vi "RSNRPZctrl.vi"(0 "VISA session in":refnum<visa-resource-name> caption="VISA resource name", 1 "Resource Name (USB::0x0aad::0x000b::100000)":string="USB::0x0aad::0x00a7::101568", 5 "RSNPRZsettings":T1 caption="Settings :", 11 "error in (no error)":errorcluster, 12 "action":enum16{"close", "update", "read", "init"}(ring)) -> (4 "dup VISA session out":refnum<visa-resource-name> caption="VISA resource name", 6 "Measurement":dbl format="%.3p", 8 "connection status":bool, 15 "error out":errorcluster)   [LabVIEW 2019]
uses:
  RSNRPZcontrol.ctl
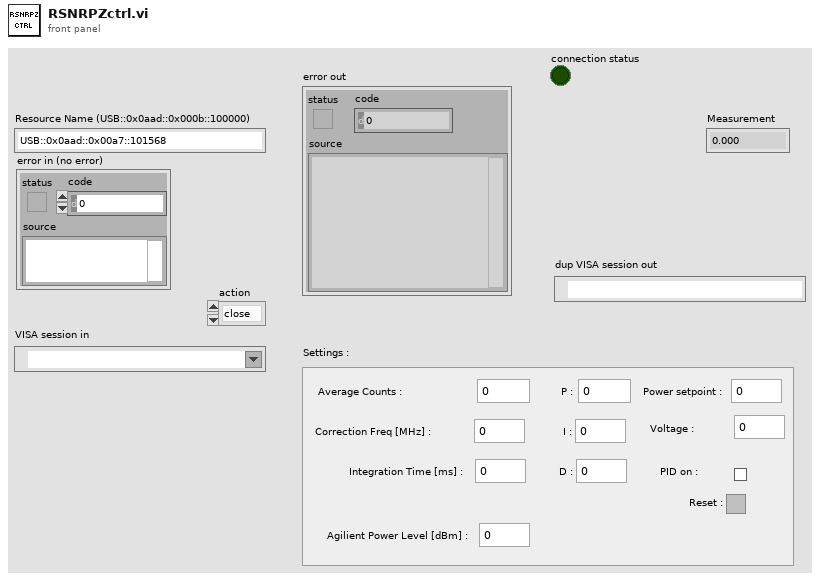
[diagram p1: front panel]
types:
  T1 = typedef "RSNRPZcontrol.ctl" = cluster{"Average Counts :":dbl, "Correction Freq [MHz] :":dbl, "Integration Time [ms] : ":dbl, "P :":dbl, "I :":dbl, "D :":dbl, "Power setpoint :":dbl, "PID on :":bool, "Voltage :":dbl, "Reset :":bool, "Agilient Power Level [dBm] :":dbl}
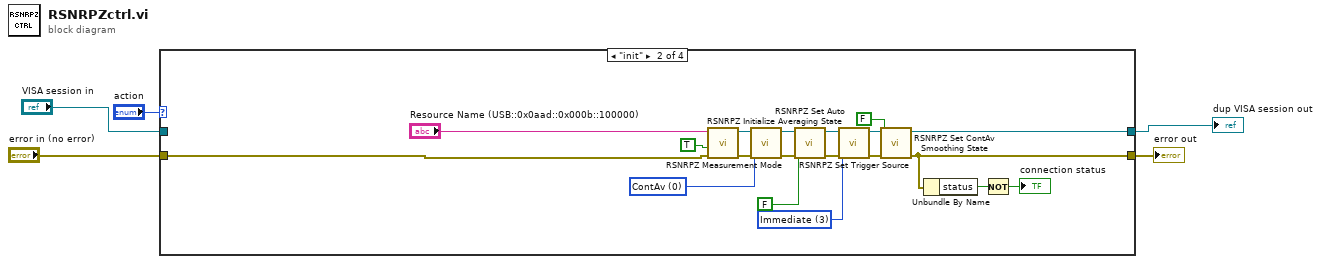
[diagram p0: block diagram]
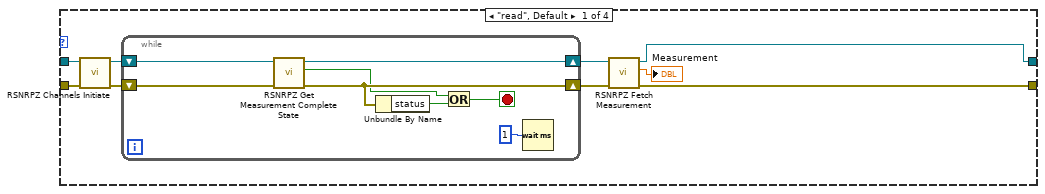
[diagram p2: hidden frame]
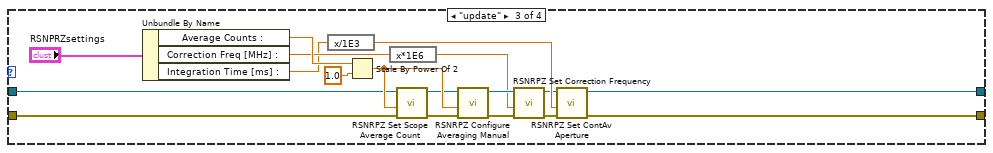
[diagram p3: hidden frame]
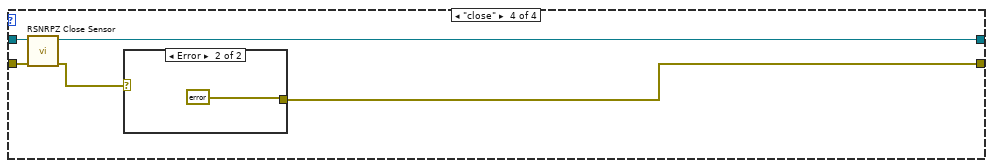
[diagram p4: hidden frame]
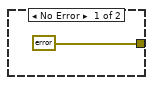
[diagram p5: hidden frame]
diagram:
  n1 = case shown="\"init\"" "action" {
    tunnel: "error in (no error)" -> [w7 w39 w59 w64]
    tunnel: [w11 w29 w46 w60] -> w3
    tunnel: [w10 w30 w48 w62] -> w2
    tunnel: "VISA session in" -> [w6 _ w47 w63]
    frame "read", Default {
      n2 = call "RSNRPZ Channels Initiate.vi"("error in (no error)"=w7, "VISA session"=w6) -> ("error out"=w14:errorcluster, "dup VISA session"=w8:refnum<visa-resource-name>)  [unwired: 8 in]
      n3 = while {
        shift-right: [w18] -> w13
        shift-left: w14 -> [w22]
        shift-right: [w21] -> w12
        shift-left: w8 -> [w20]
        stop <- w17 stop-if-true
        n4 = call "RSNRPZ Get Measurement Complete State.vi"("error in (no error)"=w22, "VISA session"=w20) -> ("error out"=w18:errorcluster, "Measurement Complete"=w15:bool, "dup VISA session"=w21:refnum<visa-resource-name>)  [unwired: 7 in]
        n5 = Unbundle By Name(w18) -> ("status"=w16:bool)
        n6 = Or(x=w15, y=w16) -> (x .or. y?=w17:bool)
        n7 = Wait (ms)(milliseconds to wait=u32 1) -> ()  [unwired: 1 out]
      }
      n8 = call "RSNRPZ Fetch Measurement.vi"("error in (no error)"=w13, "VISA session"=w12) -> ("error out"=w11:errorcluster, "Measurement"=→"Measurement":dbl, "dup VISA session"=w10:refnum<visa-resource-name>)  [unwired: 7 in]
    }
    frame "init" {
      w24 = 3 items=["Bus", "External", "Hold", "Immediate", "Internal", "External 2"] ("Trigger Source (3: Immediate)")
      w26 = 0 items=["ContAv"=0, "Buffered ContAv"=1, "Timeslot"=2, "Burst"=3, "Scope"=4, "CCDF"=6, "PDF"=7] ("Measurement Mode (ContAv)")
      n9 = call "RSNRPZ Initialize.vi"("error in (no error)"=w39, "Reset Device (T: Reset Device)"=TRUE, "Resource Name (USB::0x0aad::0x000b::100000)"="Resource Name (USB::0x0aad::0x000b::100000)") -> ("error out"=w38:errorcluster, "dup VISA session"=w37:refnum<visa-resource-name>)  [unwired: 7 in]
      n10 = call "RSNRPZ Measurement Mode.vi"("error in (no error)"=w38, "Measurement Mode (ContAv)"=w26, "VISA session"=w37) -> ("error out"=w36:errorcluster, "dup VISA session"=w33:refnum<visa-resource-name>)  [unwired: 7 in]
      n11 = call "RSNRPZ Set Auto Averaging State.vi"("error in (no error)"=w36, "Auto Enabled (On)"=FALSE, "VISA session"=w33) -> ("error out"=w35:errorcluster, "dup VISA session"=w32:refnum<visa-resource-name>)  [unwired: 7 in]
      n12 = call "RSNRPZ Set Trigger Source.vi"("error in (no error)"=w35, "Trigger Source (3: Immediate)"=w24, "VISA session"=w32) -> ("error out"=w34:errorcluster, "dup VISA session"=w31:refnum<visa-resource-name>)  [unwired: 7 in]
      n13 = call "RSNRPZ Set ContAv Smoothing State.vi"("error in (no error)"=w34, "ContAv Smoothing (T: On)"=FALSE, "VISA session"=w31) -> ("error out"=w29:errorcluster, "dup VISA session"=w30:refnum<visa-resource-name>)  [unwired: 7 in]
      n14 = Unbundle By Name(w29) -> ("status"=w27:bool)
      n15 = Not(x=w27) -> (.not. x?=→"connection status":bool)
    }
    frame "update" {
      n16 = Unbundle By Name("RSNPRZsettings") -> ("Average Counts :"=w44:dbl, "Correction Freq [MHz] :"=w43:dbl, "Integration Time [ms] :"=w42:dbl)
      n17 = expression code="x/1E3"(w42) -> (w50:dbl)
      n18 = Scale By Power Of 2(n=w44, x=1.0) -> (x*2^n=w56:dbl)
      n19 = expression code="x*1E6"(w43) -> (w52:dbl)
      n20 = call "RSNRPZ Set Scope Average Count.vi"("error in (no error)"=w59, "Count (4)"=w56, "VISA session"=w47) -> ("error out"=w57:errorcluster, "dup VISA session"=w55:refnum<visa-resource-name>)  [unwired: 7 in]
      n21 = call "RSNRPZ Configure Averaging Manual.vi"("error in (no error)"=w57, "Count (4)"=w56, "VISA session"=w55) -> ("error out"=w54:errorcluster, "dup VISA session"=w53:refnum<visa-resource-name>)  [unwired: 7 in]
      n22 = call "RSNRPZ Set Correction Frequency.vi"("error in (no error)"=w54, "Frequency ( 50.0e6 Hz)"=w52, "VISA session"=w53) -> ("error out"=w51:errorcluster, "dup VISA session"=w49:refnum<visa-resource-name>)  [unwired: 7 in]
      n23 = call "RSNRPZ Set ContAv Aperture.vi"("error in (no error)"=w51, "ContAv Aperture (0.02 s)"=w50, "VISA session"=w49) -> ("error out"=w46:errorcluster, "dup VISA session"=w48:refnum<visa-resource-name>)  [unwired: 7 in]
    }
    frame "close" {
      n24 = call "RSNRPZ Close Sensor.vi"("error in (no error)"=w64, "VISA session"=w63) -> ("error out"=w61:errorcluster, "dup VISA session"=w62:refnum<visa-resource-name>)  [unwired: 8 in]
      n25 = case shown="Error" w61 {
        tunnel: [errorcluster {"status"=FALSE, "code"=0, "source"=""} ("error out") errorcluster {"status"=FALSE, "code"=0, "source"=""} ("error out")] -> w60
        frame No Error {
        }
        frame Error {
        }
      }
    }
  }
  "error out" <- w3
  "dup VISA session out" <- w2
